vi "Write multi.vi"(0 "tdms file in":refnum<k34>, 5 "group":string, 7 "Channel":string[](array[string]), 9 "Data":dbl[](array[numeric]), 11 "error in (no error)":errorcluster) -> (4 "tdms file out":refnum<k34>, 6 "group 2":string, 8 "Channel 2":string[](array[string]), 15 "error out":errorcluster)   [LabVIEW 2013, in "Scale.lvlib" / "Scale.lvclass"]
uses:
  Scale.lvclass
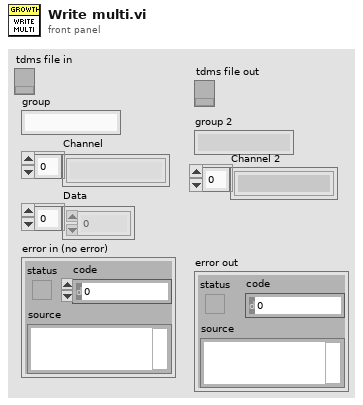
[diagram p1: front panel]
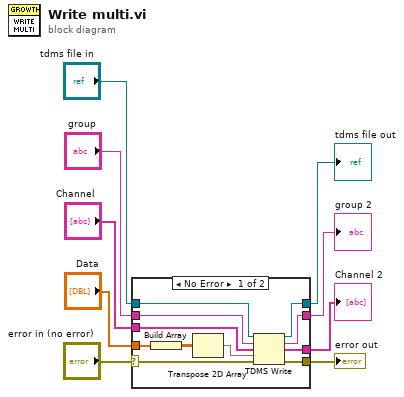
[diagram p0: block diagram]
diagram:
  n1 = case shown="No Error" "error in (no error)" {
    selector: "error in (no error)" -> [w10 w23]
    tunnel: "tdms file in" -> [w13 w24]
    tunnel: "group" -> [w20 w22]
    tunnel: "Channel" -> [w19 w21]
    tunnel: [w12 w24] -> w2
    tunnel: [w11 w23] -> w7
    tunnel: "Data" -> [w18 _]
    tunnel: [w15 w22] -> w4
    tunnel: [w14 w21] -> w3
    frame No Error {
      n2 = Build Array(w18) -> (w17:dbl[][])
      n3 = Transpose 2D Array(2D array=w17) -> (transposed array=w16:dbl[][])
      n4 = TDMS Write(0:w13, 5:w20, 7:w19, 9:w16, 11:w10) -> (4:w12:refnum<k34>, 6:w15:string, 8:w14:string[], 15:w11:errorcluster)  [unwired: 1 in]
    }
    frame Error {
    }
  }
  "error out" <- w7
  "group 2" <- w4
  "Channel 2" <- w3
  "tdms file out" <- w2
